vi "CheckCollisionShipInvader.vi"(8 "ShipRectangle":T1, 11 "InvaderRectangle":T1) -> (3 "Collision":bool)   [LabVIEW 2019]
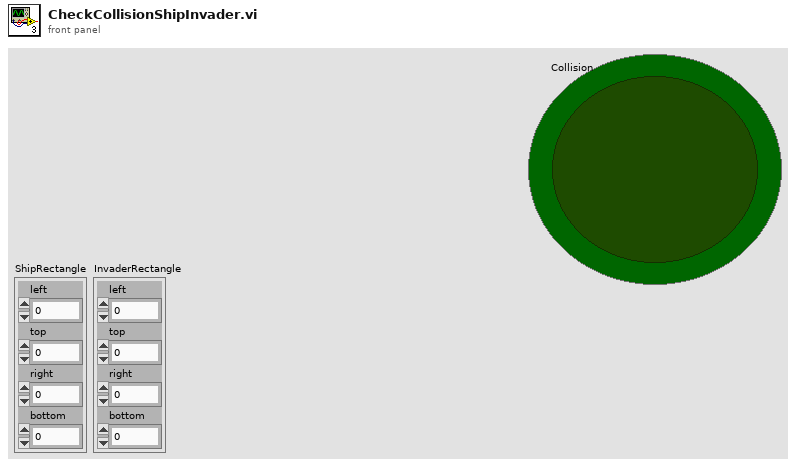
[diagram p1: front panel]
types:
  T1 = cluster{"left":i16, "top":i16, "right":i16, "bottom":i16}
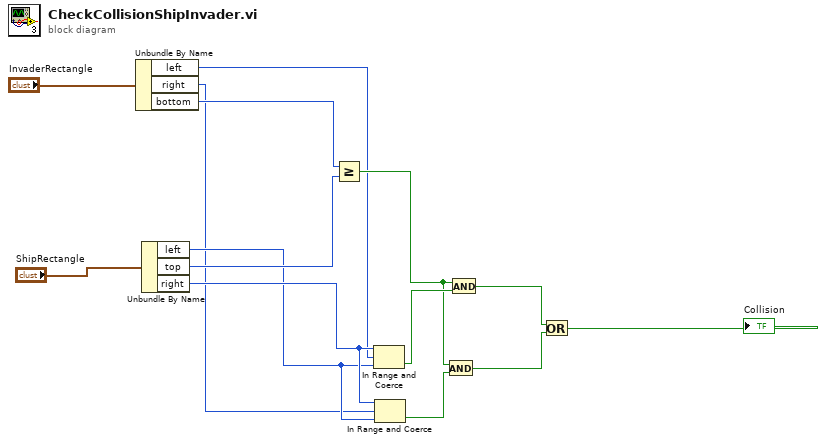
[diagram p0: block diagram]
diagram:
  n1 = Unbundle By Name("InvaderRectangle") -> ("left"=w5:i16, "right"=w4:i16, "bottom"=w12:i16)
  n2 = Unbundle By Name("ShipRectangle") -> ("left"=w9:i16, "top"=w11:i16, "right"=w10:i16)
  n3 = Greater Or Equal?(x=w12, y=w11) -> (x >= y?=w7:bool)
  n4 = In Range and Coerce(upper limit=w10, x=w5, lower limit=w9) -> (In Range?=w8:bool)  [unwired: 1 out]
  n5 = In Range and Coerce(upper limit=w10, x=w4, lower limit=w9) -> (In Range?=w6:bool)  [unwired: 1 out]
  n6 = And(x=w7, y=w6) -> (x .and. y?=w2:bool)
  n7 = And(x=w7, y=w8) -> (x .and. y?=w3:bool)
  n8 = Or(x=w3, y=w2) -> (x .or. y?=→"Collision":bool)
